vi "set32bitIntegerArray.vi"(11 "inI32Array":i32[](array[numeric])) -> ()   [LabVIEW 2014]
uses:
  GlobalVariables.vi
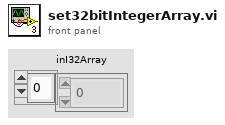
[diagram p1: front panel]
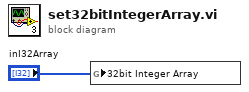
[diagram p0: block diagram]
diagram:
  n1 = global write "GlobalVariables.vi" "32bit Integer Array"("inI32Array") -> ()
